vi "DDAQ-Set.vi"(8 "error in (no error)":errorcluster, 9 "Set Value":string, 10 "SCPI-like Keyword (leave off space, value)":string, 11 "connection ID":refnum<k5>) -> (0 "error out":errorcluster, 3 "connection ID out":refnum<k5>)   [LabVIEW 2020]
panel:
  out "bytes written":i32
  out "Command":string
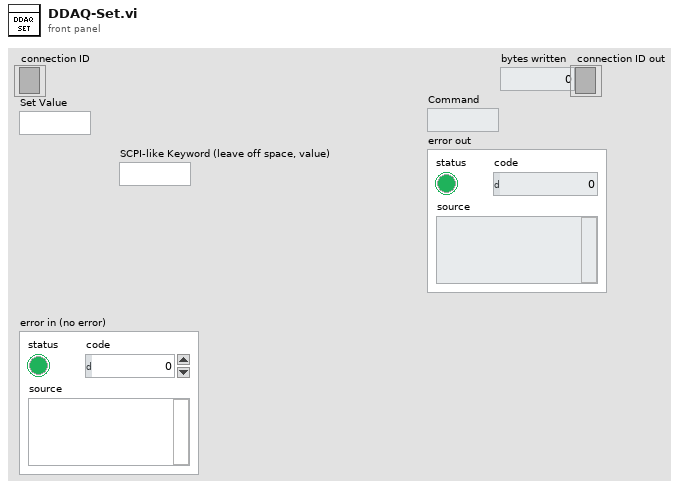
[diagram p1: front panel]
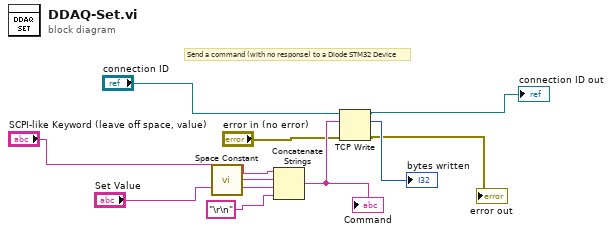
[diagram p0: block diagram]
diagram:
  # "Send a command (with no response) to a Diode STM32 Device"
  n1 = call <vilib>:"Space Constant.vi"() -> ("String"=w2:string)
  n2 = Concatenate Strings("SCPI-like Keyword (leave off space, value)", w2, "Set Value", "\r\n") -> (w9:string)
  "Command" <- w9
  n3 = TCP Write(connection ID="connection ID", data in=w9, error in (no error)="error in (no error)") -> (connection ID out=→"connection ID out":refnum<k5>, bytes written=→"bytes written":i32, error out=→"error out":errorcluster)  [unwired: 1 in]
